vi "Pack for gRPC.vi"(8 "error in":errorcluster, 9 "configuration / results":enum16{"Configuration", "Results"}(ring), 10 "data value":variant, 11 "measurement customizations in":refnum<class "Measurement Plugin.lvclass">) -> (0 "error out":errorcluster, 2 "any":T1, 3 "measurement customizations out":refnum<class "Measurement Plugin.lvclass">)   [LabVIEW 2021, in "channelGanging.lvlib" / "Measurement Plugin.lvclass"]
uses:
  Measurement Plugin.lvclass
  Measurement Plugin.lvclass/Measurement Plugin.ctl
  Measurement Configuration.ctl
  channelGanging.lvlib
  Measurement Results.ctl
  a6012965-5700-4384-8228-972e71b6560c.vi
  2eca732d-dbaa-43bf-a7dd-ede2da65bc1b.vi
  <vilib>/MeasurementLink/MeasurementLink Measurement Server/Measurement Plugin Service/Measurement Plugin Service.lvclass
  C:/Program Files/National Instruments/LabVIEW 2021/vi.lib/MeasurementLink/MeasurementLink Measurement Server/Measurement Plugin Service/Measurement Plugin Service.lvclass
  C:/Users/Administrator/Documents/GitHub/pmic-labview/source/measurements/channelGanging/channelGanging/Advanced/Measurement Plugin.lvclass
  <vilib>/gRPC/LabVIEW gRPC Library/Shared/Any.ctl
  <vilib>/gRPC/LabVIEW gRPC Library/grpc-lvsupport-release.lvlib
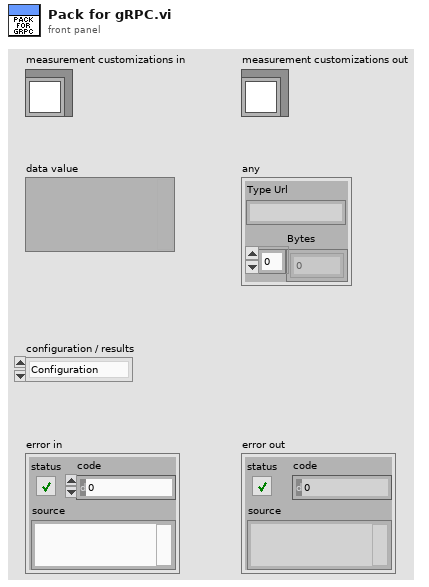
[diagram p1: front panel]
types:
  T1 = typedef "grpc-lvsupport-release.lvlib/Any.ctl" = cluster{"Type Url":string, "Bytes":u8[]}
  T2 = typedef "grpc-lvsupport-release.lvlib/grpcId.ctl" = u64
  T3 = typedef "channelGanging.lvlib/Measurement Configuration.ctl" = cluster{"Source channel names":i32[], "Source resource names":string[], "Source channel mode":enum32{"Master", "Slave", "Slave- inverted"}[], "Source system configuration":enum32{"Parallel", "Series"}, "Source voltage level":dbl, "Source voltage level range":dbl, "Source sense":enum32{"Remote", "Local"}, "Source limit symmetry":enum32{"Asymmetric", "Symmetric"}, "Source current limit range":dbl, "Source current limit low":dbl, "Source current limit high":dbl, "Source aperture time":dbl, "Source transient response":enum32{"Fast", "Normal", "Slow"}, "Load channel names":i32[], "Load resource names":string[], "Load channel mode":enum32{"Master", "Slave", "Slave- inverted"}[], "Load system configuration":enum32{"Parallel", "Series"}, "Load current Level":dbl, "Load current level range":dbl, "Load Sense":enum32{"Remote", "Local"}, "Load limit symmetry":enum32{"Asymmetric", "Symmetric"}, "Load voltage limit range":dbl, "Load voltage limit low":dbl, "Load voltage limit high":dbl, "Load aperture time":dbl, "Load transient response":enum32{"Fast", "Normal", "Slow"}, "Measurement time":dbl}
  T4 = typedef "channelGanging.lvlib/Measurement Results.ctl" = cluster{"dt 2":dbl, "Source voltages":dbl[], "Source currents":dbl[], "Load voltages":dbl[], "Load currents":dbl[]}
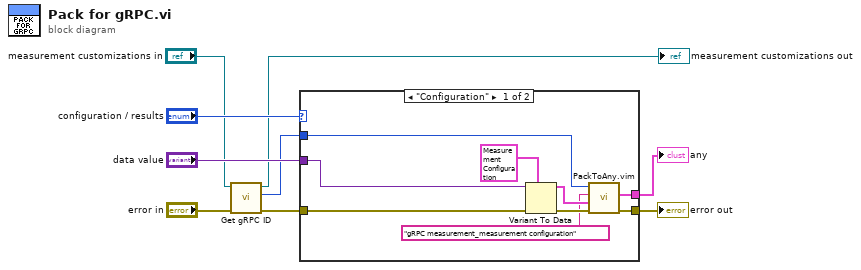
[diagram p0: block diagram]
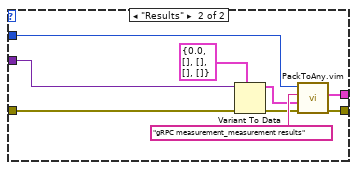
[diagram p2: hidden frame]
diagram:
  n1 = call <vilib>:"Get gRPC ID.vi"("error in"="error in", "measurement plugin service in"="measurement customizations in") -> ("error out"=w4:errorcluster, "gRPC ID"=w1:T2, "measurement plugin service out"=→"measurement customizations out":refnum<class "Measurement Plugin.lvclass">)  [unwired: 7 in]
  n2 = case shown="\"Configuration\"" "configuration / results" {
    tunnel: w4 -> [w18 w27]
    tunnel: "data value" -> [w17 w26]
    tunnel: w1 -> [w14 w22]
    tunnel: [w16 w24] -> w8
    tunnel: [w15 w23] -> w7
    frame "Configuration" {
      n3 = Variant To Data(error in=w18, type=T3 {"Source channel names"=[], "Source resource names"=[], "Source channel mode"=[], "Source system configuration"=enum."Parallel", "Source voltage level"=2.0, "Source voltage level range"=20.0, "Source sense"=enum."Remote", "Source limit symmetry"=enum."Asymmetric", "Source current limit range"=2.0, "Source current limit low"=2.0, "Source current limit high"=20.0, "Source aperture time"=0.01, "Source transient response"=enum."Slow", "Load channel names"=[], "Load resource names"=[], "Load channel mode"=[], "Load system configuration"=enum."Parallel", "Load current Level"=2.0, "Load current level range"=20.0, "Load Sense"=enum."Remote", "Load limit symmetry"=enum."Asymmetric", "Load voltage limit range"=2.0, "Load voltage limit low"=2.0, "Load voltage limit high"=20.0, "Load aperture time"=0.01, "Load transient response"=enum."Slow", "Measurement time"=0.01} ("measurement configuration"), Variant=w17) -> (data=w13:T3, error out=w12:errorcluster)
      n4 = call "PackToAny.vim"("error in"=w12, "Data To Pack"=w13, "Message Type"="gRPC measurement_measurement configuration", "gRPCid in"=w14) -> ("error out"=w16:errorcluster, "Any"=w15:T1)  [unwired: 5 in, 1 out]
    }
    frame "Results" {
      n5 = Variant To Data(error in=w27, type=T4 {"dt 2"=0.0, "Source voltages"=[], "Source currents"=[], "Load voltages"=[], "Load currents"=[]} ("Measurement Results"), Variant=w26) -> (data=w20:T4, error out=w19:errorcluster)
      n6 = call "PackToAny.vim"("error in"=w19, "Data To Pack"=w20, "Message Type"="gRPC measurement_measurement results", "gRPCid in"=w22) -> ("error out"=w24:errorcluster, "Any"=w23:T1)  [unwired: 5 in, 1 out]
    }
  }
  "error out" <- w8
  "any" <- w7
